vi "test_deltaF.vi"() -> ()   [LabVIEW 2013]
panel:
  out "I":dbl[](array[numeric])
  out "dbl precision":dbl[](array[numeric])
  out "Q in":fxp<+/-,16,14>[](array[numeric])
  out "Waveform Graph":dbl[][](graph)
  out "Q out":fxp<+/-,16,14>[](array[numeric])
  out "deltaF":fxp<+/-,32,30>[](array[numeric])
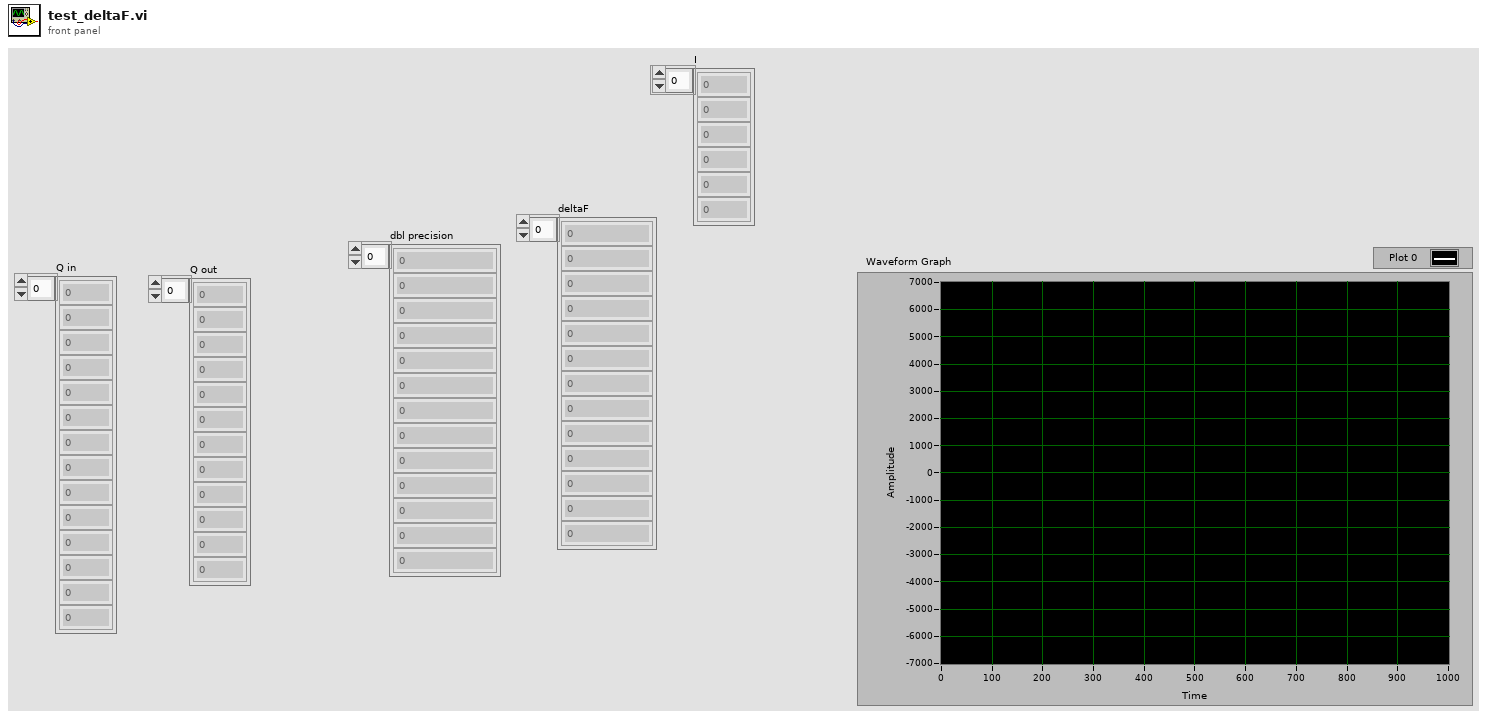
[diagram p1: front panel]
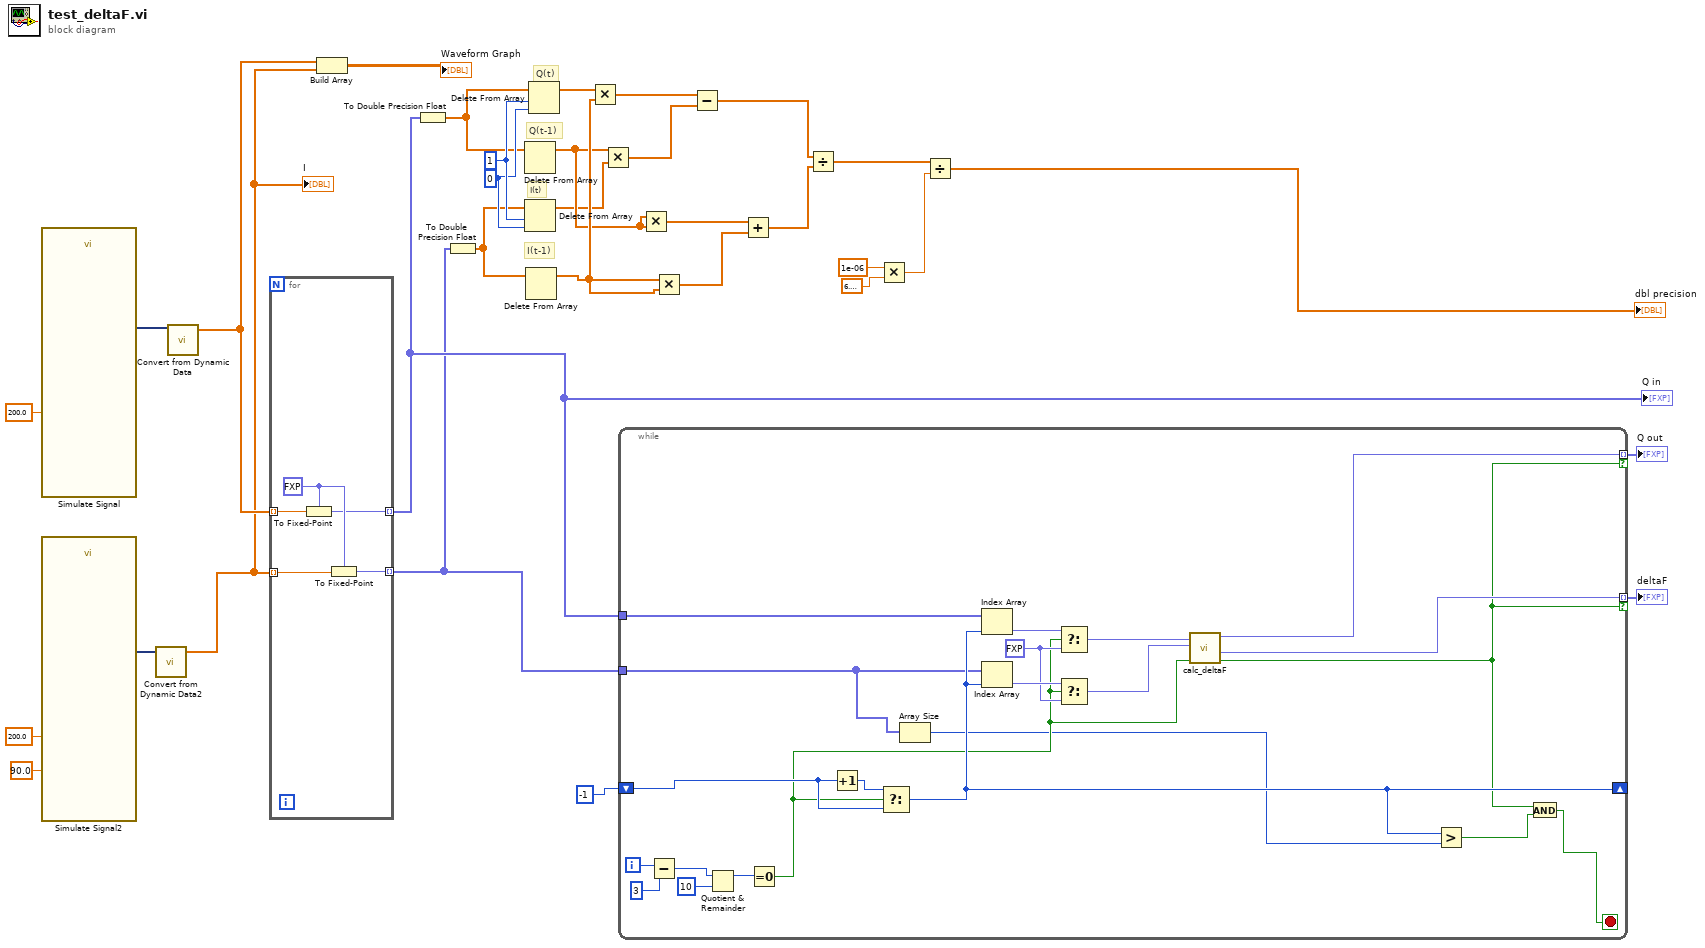
[diagram p0: block diagram]
diagram:
  w7 = 0 ("index")
  w8 = 1 ("length")
  # "I(t-1)"
  # "I(t)"
  # "Q(t-1)"
  # "Q(t)"
  n1 = call "Simulate Signal"("Noise amplitude"=200.0) -> ("Sine with Uniform Noise"=w29:dynamicdata)  [unwired: 13 in, 1 out]
  n2 = call "Simulate Signal2"("Phase"=90.0, "Noise amplitude"=200.0) -> ("Sine with Uniform Noise"=w27:dynamicdata)  [unwired: 12 in, 1 out]
  n3 = call "Convert from Dynamic Data2"("Dynamic Data Type"=w27) -> ("Array"=w21:dbl[])  [unwired: 3 in]
  "I" <- w21
  n4 = call "Convert from Dynamic Data"("Dynamic Data Type"=w29) -> ("Array"=w22:dbl[])  [unwired: 3 in]
  n5 = for {
    tunnel: w21 -> [w36] mode=indexing
    tunnel: w22 -> [w37] mode=indexing
    tunnel: [w34] -> w6 mode=indexing
    tunnel: [w33] -> w4 mode=indexing
    w35 = fxp<+/-,16,14> 0.0 ("f")
    n6 = To Fixed-Point(fixed-point type=w35, number=w37) -> (fixed-point=w34:fxp<+/-,16,14>)
    n7 = To Fixed-Point(fixed-point type=w35, number=w36) -> (fixed-point=w33:fxp<+/-,16,14>)
  }
  "Q in" <- w6
  n8 = Build Array(w22, w21) -> (→"Waveform Graph":dbl[][])
  n9 = To Double Precision Float(number=w6) -> (double precision float=w5:dbl[])
  n10 = To Double Precision Float(number=w4) -> (double precision float=w3:dbl[])
  n11 = Delete From Array(array=w5) -> (array with subset deleted=w17:dbl[])  [unwired: 2 in, 1 out]
  n12 = Delete From Array(array=w3, length=w8, index=w7) -> (array with subset deleted=w9:dbl[])  [unwired: 1 out]
  n13 = Delete From Array(array=w3) -> (array with subset deleted=w18:dbl[])  [unwired: 2 in, 1 out]
  n14 = Delete From Array(array=w5, length=w8, index=w7) -> (array with subset deleted=w25:dbl[])  [unwired: 1 out]
  n15 = Multiply(x=w25, y=w18) -> (x*y=w24:dbl[])
  n16 = Multiply(x=w17, y=w9) -> (x*y=w23:dbl[])
  n17 = while {
    tunnel: w6 -> [w52]
    shift-right: [w55] -> _
    shift-left: -1 ("y") -> [w56]
    tunnel: w4 -> [w41]
    tunnel: [w43] -> w30 mode=indexing if=w39
    tunnel: [w42] -> w31 mode=indexing if=w39
    i -> [w51]
    stop <- w46 stop-if-true
    w48 = fxp<+/-,16,14> 0.0 ("f")
    n18 = Subtract(x=w51, y=3) -> (x-y=w49:i32)
    n19 = Quotient & Remainder(x=w49, y=10) -> (x-y*floor(x/y)=w58:i32)  [unwired: 1 out]
    n20 = Equal To 0?(x=w58) -> (x = 0?=w44:bool)
    n21 = Increment(x=w56) -> (x+1=w57:i32)
    n22 = Select(t=w57, s=w44, f=w56) -> (s? t:f=w55:i32)
    n23 = Array Size(array=w41) -> (size(s)=w40:i32)
    n24 = Index Array(array=w52, index=w55) -> (element=w53:fxp<+/-,16,14>)
    n25 = Index Array(array=w41, index=w55) -> (element=w54:fxp<+/-,16,14>)
    n26 = Select(t=w53, s=w44, f=w48) -> (s? t:f=w38:fxp<+/-,16,14>)
    n27 = Select(t=w54, s=w44, f=w48) -> (s? t:f=w45:fxp<+/-,16,14>)
    n28 = call "calc_deltaF.vi"("valid in"=w44, "Q in"=w45, "I in"=w38) -> ("output valid"=w39:bool, "delta_F"=w42:fxp<+/-,32,30>, "I out"=w43:fxp<+/-,16,14>)  [unwired: 5 in, 1 out]
    n29 = Greater?(x=w55, y=w40) -> (0:w47:bool)
    n30 = And(x=w39, y=w47) -> (x .and. y?=w46:bool)
  }
  "deltaF" <- w31
  "Q out" <- w30
  n31 = Multiply(x=w17, y=w17) -> (x*y=w19:dbl[])
  n32 = Multiply(x=w18, y=w18) -> (x*y=w20:dbl[])
  n33 = Subtract(x=w24, y=w23) -> (x-y=w16:dbl[])
  n34 = Add(x=w19, y=w20) -> (x+y=w15:dbl[])
  n35 = Divide(x=w16, y=w15) -> (x/y=w11:dbl[])
  n36 = Multiply(x=1e-06, y=6.283185307179586) -> (x*y=w12:dbl)
  n37 = Divide(x=w11, y=w12) -> (x/y=→"dbl precision":dbl[])
